vi "Evaluate Part 2.vi"() -> ()   [LabVIEW 2021]
uses:
  Proto/Proto.lvclass
panel:
  out "Sum":u64
  in  "Input":string="rn=1,cm-,qp=3,cm=2,qp-,pc=4,ot=9,ab=5,pc-,pc=6,ot=7"
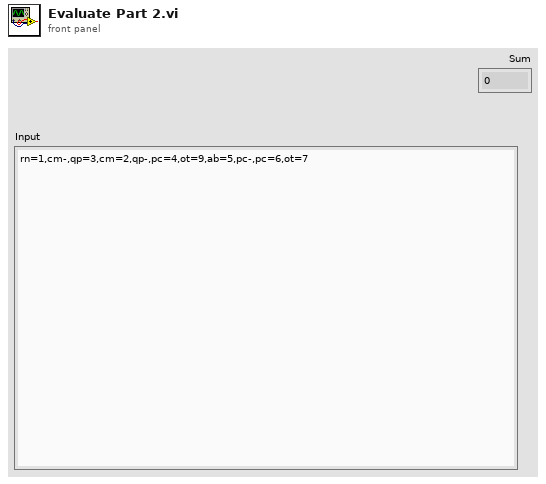
[diagram p1: front panel]
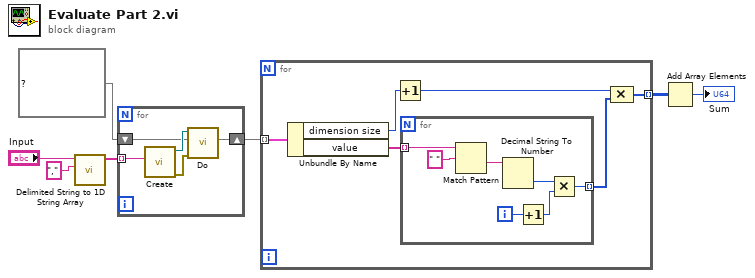
[diagram p0: block diagram]
diagram:
  n1 = call <vilib>:"Delimited String to 1D String Array.vi"("delimiter"=",", "delimited string"="Input") -> ("string array"=w5:string[])  [unwired: 9 in]
  n2 = for {
    tunnel: w5 -> [w12] mode=indexing
    shift-right: [w8] -> w2
    shift-left: map{i32, string[]} {} ("Boxes") -> [w9]
    n3 = call "Create.vi"("Input"=w12) -> ("error out"=w10:errorcluster, "Proto"=w11:refnum<class "Proto.lvclass">)  [unwired: 9 in]
    n4 = call "Do.vi"("error in (no error)"=w10, "Boxes"=w9, "Proto in"=w11) -> ("Boxes out"=w8:map{i32, string[]})  [unwired: 6 in, 2 out]
  }
  n5 = for {
    tunnel: w2 -> [w18] mode=indexing
    tunnel: [w13] -> w1 mode=indexing
    n6 = Unbundle By Name(w18) -> ("dimension size"=w17:i32, "value"=w15:string[])
    n7 = Increment(x=w17) -> (x+1=w16:i32)
    n8 = for {
      tunnel: w15 -> [w23] mode=indexing
      tunnel: [w19] -> w14 mode=indexing
      i -> [w25]
      n9 = Match Pattern(string=w23, regular expression=" " ("string")) -> (after substring=w21:string)  [unwired: 1 in, 3 out]
      n10 = Decimal String To Number(string=w21) -> (number=w20:i32)  [unwired: 2 in, 1 out]
      n11 = Increment(x=w25) -> (x+1=w24:i32)
      n12 = Multiply(x=w20, y=w24) -> (x*y=w19:i32)
    }
    n13 = Compound Arithmetic op=MULTIPLY(w16, w14) -> (w13:i32[])
  }
  n14 = Add Array Elements(numeric array=w1) -> (sum=→"Sum":i32)
